vi "Percentage Drive.vi"(8 "error in (no error)":errorcluster, 9 "Right Percent":dbl, 10 "Left Percent":dbl, 11 "Tank Drive in":refnum<class "Tank Drive.lvclass">) -> (0 "error out":errorcluster, 3 "Tank Drive out":refnum<class "Tank Drive.lvclass">)   [LabVIEW 2019, in "Drive.lvlib" / "Tank Drive.lvclass"]
doc: "switches into percent vbus drive"
uses:
  Tank Drive.lvclass
  Controls/Drive State.ctl
  Tank Drive.lvclass/Tank Drive.ctl
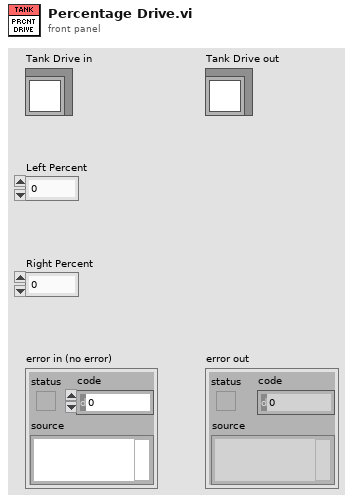
[diagram p1: front panel]
types:
  T1 = typedef "Drive.lvlib/Tank Drive.lvclass/Drive State.ctl" = enum16{"Percentage Drive", "Velocity Drive", "PID to Position", "Motion Profile"}
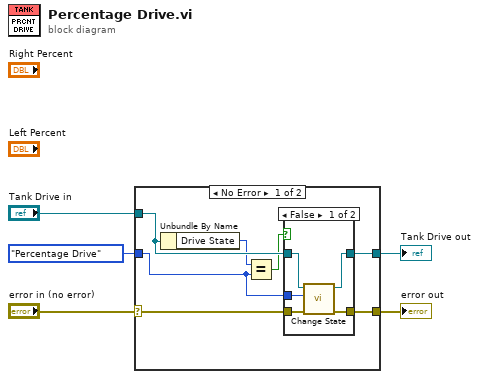
[diagram p0: block diagram]
diagram:
  n1 = case shown="No Error" "error in (no error)" {
    selector: "error in (no error)" -> [w11 w21]
    tunnel: [w10 w21] -> w4
    tunnel: [w9 w20] -> w2
    tunnel: "Tank Drive in" -> [w12 w20]
    tunnel: Drive_State."Percentage Drive" ("New State") -> [w7 _]
    frame No Error {
      n2 = Unbundle By Name(w12) -> ("Drive State"=w8:T1)
      n3 = Equal?(x=w8, y=w7) -> (x = y?=w6:bool)
      n4 = case shown="False" w6 {
        tunnel: w12 -> [w17 w19]
        tunnel: w11 -> [w16 w18]
        tunnel: [w15 w18] -> w10
        tunnel: [w14 w19] -> w9
        tunnel: w7 -> [w13 _]
        frame False {
          n5 = call-dynamic "Change State.vi"("error in (no error)"=w16, "New State"=w13, "Tank Drive in"=w17) -> ("error out"=w15:errorcluster, "Tank Drive out"=w14:refnum<class "Tank Drive.lvclass">)  [unwired: 7 in]
        }
        frame True {
        }
      }
    }
    frame Error {
    }
  }
  "error out" <- w4
  "Tank Drive out" <- w2
